vi "Data Read Single.vi"(0 "VISA resource name":refnum<visa-resource-name>, 1 "Source (0: Function)":u16(ring) items=["Function", "Calculation 1", "Calculation 2", "Calculation 3"], 5 "error in (no error)":errorcluster, 8 "Timeout (25000 ms)":u32=25000) -> (14 "VISA resource name out":refnum<visa-resource-name>, 15 "Measurement":dbl, 16 "Channel":i32, 17 "Units":string, 19 "error out":errorcluster)   [LabVIEW 2016, in "Keithley 2000.lvlib"]
doc: "This VI reads a measurement or calculation from the instrument. It also returns the channel number and units of the measurement (if applicable)."
uses:
  Keithley 2000.lvlib
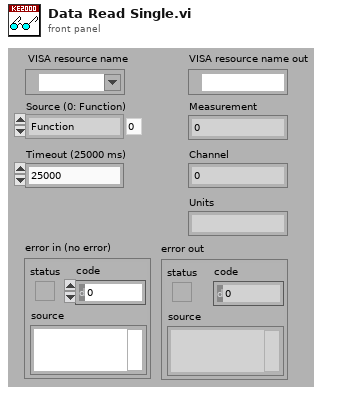
[diagram p1: front panel]
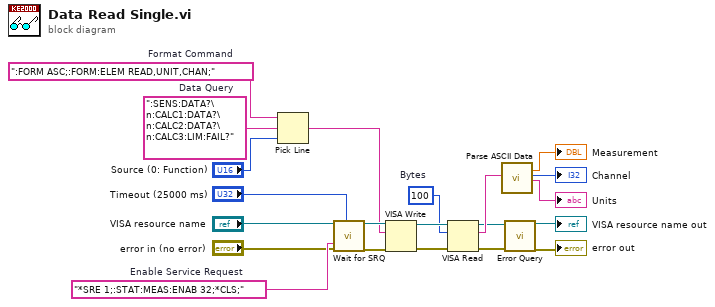
[diagram p0: block diagram]
diagram:
  w11 = ":SENS:DATA?\n:CALC1:DATA?\n:CALC2:DATA?\n:CALC3:LIM:FAIL?"  # Data Query
  w12 = ":FORM ASC;:FORM:ELEM READ,UNIT,CHAN;"  # Format Command
  w3 = "*SRE 1;:STAT:MEAS:ENAB 32;*CLS;"  # Enable Service Request
  w19 = u32 100  # Bytes
  n1 = Pick Line(string ("")=w12, multi-line string=w11, line index="Source (0: Function)") -> (output string=w9:string)
  n2 = call "Wait for SRQ.vi"("VISA resource name"="VISA resource name", "SRQ Enable Command"=w3, "error in (no error)"="error in (no error)", "Timeout (25000 ms)"="Timeout (25000 ms)") -> ("VISA resource name out"=w13:refnum<visa-resource-name>, "error out"=w14:errorcluster)  [unwired: 14 in]
  n3 = VISA Write(VISA resource name=w13, write buffer=w9, error in (no error)=w14) -> (VISA resource name out=w20:refnum<visa-resource-name>, error out=w21:errorcluster)  [unwired: 1 out]
  n4 = VISA Read(VISA resource name=w20, byte count=w19, error in (no error)=w21) -> (VISA resource name out=w7:refnum<visa-resource-name>, read buffer=w18:string, error out=w6:errorcluster)  [unwired: 1 out]
  n5 = call "Parse ASCII Data.vi"("ASCII Data (Empty)"=w18) -> ("Measurement"=→"Measurement":dbl, "Channel"=→"Channel":i32, "Units"=→"Units":string)  [unwired: 16 in]
  n6 = call "Error Query.vi"("VISA resource name"=w7, "error in (no error)"=w6) -> ("VISA resource name out"=→"VISA resource name out":refnum<visa-resource-name>, "error out"=→"error out":errorcluster)  [unwired: 14 in, 2 out]
